vi "ColorSmartCheck.vi"() -> ()   [LabVIEW 2018]
uses:
  <vilib>/myRIO/Instrument Drivers/Onboard IO/AI/typedefs/AI Reference.ctl
  <vilib>/myRIO/Common/Instrument Driver Framework/Utilities/typedefs/myRIO Generic Hardware Reference.ctl
  <vilib>/myRIO/Common/Instrument Driver Framework/Utilities/typedefs/Hardware Version Enum.ctl
  <vilib>/myRIO/Common/Instrument Driver Framework/Utilities/typedefs/myRIO v1.0 Reference.ctl
  <vilib>/myRIO/Common/Instrument Driver Framework/Utilities/typedefs/Generic FPGA Reference.ctl
  <vilib>/myRIO/Common/Instrument Driver Framework/myRIO v1.0/AI/typedefs/AI Channels List.ctl
  <vilib>/myRIO/Common/Instrument Driver Framework/myRIO v1.0/AI/typedefs/AI Channels Enum.ctl
  <vilib>/myRIO/Common/Instrument Driver Framework/Utilities/typedefs/Analog Scaling Constants List.ctl
  <vilib>/myRIO/Common/Instrument Driver Framework/Utilities/typedefs/Analog Scaling Constants.ctl
  <vilib>/userdefined/High Color/nirio_resource_hc.ctl
  <vilib>/Analysis/coordinate.llb/2D Cartesian Coordinate Rotation (Scalar).vi
  <vilib>/Analysis/coordinate.llb/2D Cartesian Coordinate Shift (Scalar).vi
  <vilib>/myRIO/Common/Instrument Driver Framework/Utilities/vis/Is FPGA Ref Available.vi
  <vilib>/myRIO/Common/Instrument Driver Framework/myRIO v1.0/AI/vis/myRIO v1.1 Open AI.vi
  <vilib>/myRIO/Instrument Drivers/Onboard IO/AI/vis/Read.vi
  <vilib>/myRIO/Common/Instrument Driver Framework/Utilities/vis/Validate Channels.vi
  <vilib>/myRIO/Common/Instrument Driver Framework/myRIO v1.0/AI/vis/myRIO v1.0 Reserve AI.vi
  <vilib>/myRIO/Common/Instrument Driver Framework/myRIO v1.0/AI/vis/myRIO v1.0 Build MUX Configuration AI.vi
  <vilib>/myRIO/Common/Instrument Driver Framework/myRIO v1.0/Resource Manager/vis/myRIO v1.0 Reserve Channel List.vi
  <vilib>/myRIO/Common/Instrument Driver Framework/myRIO v1.0/Resource Manager/vis/myRIO v1.0 Reserve Channel.vi
  <vilib>/myRIO/Common/Instrument Driver Framework/myRIO v1.0/Resource Manager/vis/myRIO v1.0 Unreserve Channel.vi
  <vilib>/myRIO/Common/Instrument Driver Framework/myRIO v1.0/Resource Manager/vis/myRIO v1.0 Build Mutex Name.vi
  <vilib>/Utility/VariantDataType/GetNumericInfo.vi
  <vilib>/Utility/error.llb/Error Cluster From Error Code.vi
  <vilib>/myRIO/Common/Instrument Driver Framework/myRIO v1.0/myRIO v1.1 Open.vi
  <vilib>/myRIO/Common/Instrument Driver Framework/myRIO v1.0/AI/vis/myRIO v1.0 Get Scaling Constants AI.vi
  <vilib>/myRIO/Common/Instrument Driver Framework/Utilities/vis/IO Manager.vi
  <vilib>/myRIO/Common/Instrument Driver Framework/Utilities/vis/Configuration Manager.vi
  <vilib>/myRIO/Common/Instrument Driver Framework/myRIO v1.0/myRIO v1.0 Close.vi
  <vilib>/myRIO/Common/Instrument Driver Framework/myRIO v1.0/AI/vis/myRIO v1.0 Read AI.vi
  <vilib>/myRIO/Express VI/Onboard IO/AI/AI Express VI.xnode
  <vilib>/myRIO/Instrument Drivers/Onboard IO/AI/vis/myRIO AI Open.xnode
  <vilib>/myRIO/Instrument Drivers/Onboard IO/AI/AI.lvlib
  <vilib>/Analysis/NI_AALPro.lvlib
panel:
  out "element":string
  out "Found":bool
  out "B/AI0 (Pin 3) 2":dbl
  in  "Theta":dbl
  in  "Right Arm":bool
  in  "Position 2":cluster{"X":dbl, "Y":dbl, "Theta":dbl}
  out "B/AI0 (Pin 3)":dbl
  out "Position":cluster{"X":dbl, "Y":dbl, "Theta":dbl}
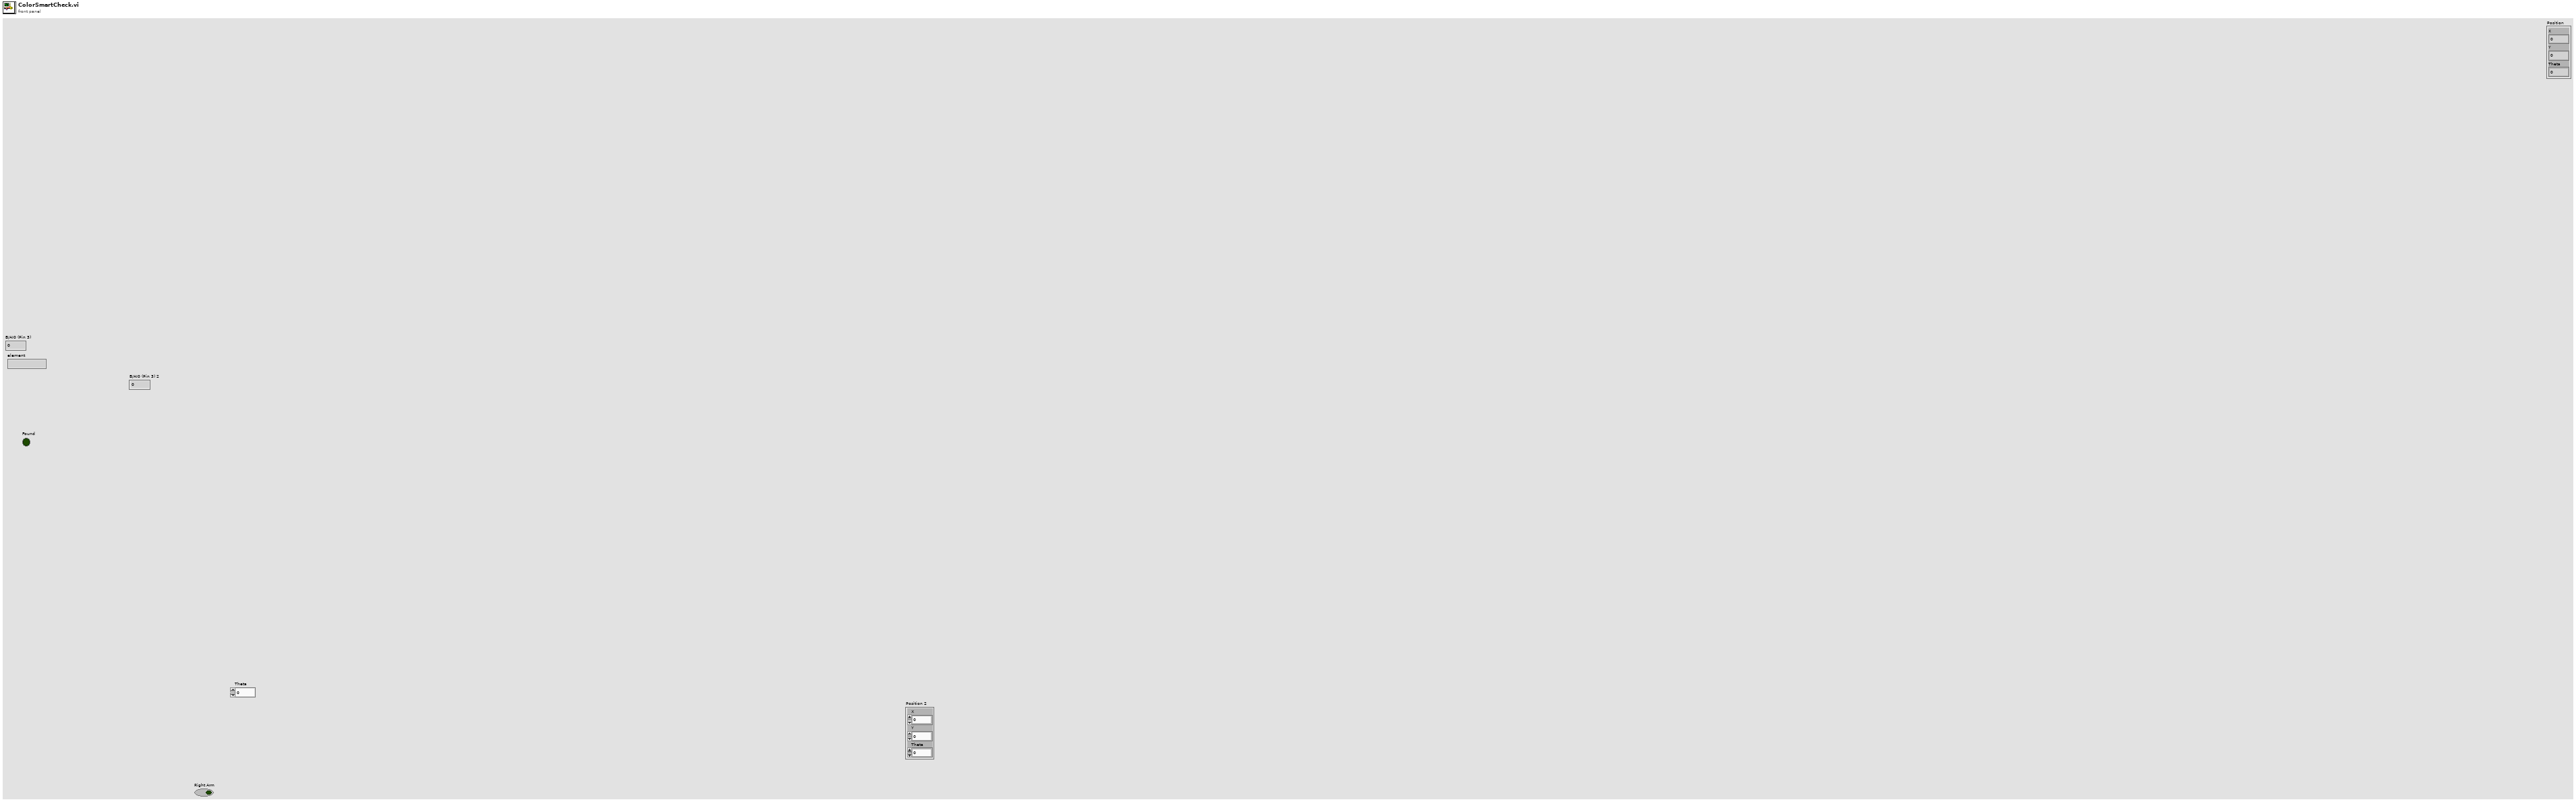
[diagram p1: front panel]
types:
  T1 = typedef "AI.lvlib/AI Reference.ctl" = cluster{"myRIO Reference":T2, "AI Channels List":T6, "AI Scaling Constants List":T8}
  T2 = typedef "myRIO Generic Hardware Reference.ctl" = cluster{"myRIO Model":T3, "myRIO Hardware Reference":T4}
  T3 = typedef "Hardware Version Enum.ctl" = enum16{"Unknown", "myRIO-1900", "myRIO-1950", "roboRIO", "NI ELVIS RIO CM", "ELVIS III"}
  T4 = typedef "myRIO v1.0 Reference.ctl" = cluster{"Generic FPGA Reference":T5, "Allow multiple opens":bool}
  T5 = typedef "Generic FPGA Reference.ctl" = refnum<k20>
  T6 = typedef "AI Channels List.ctl" = T7[]
  T7 = typedef "AI Channels Enum.ctl" = enum16{"Not Connected", "AudioIn/Left", "AudioIn/Right", "C/AI0", "C/AI1", "A/AI0", "A/AI1", "A/AI2", "A/AI3", "A/AI4", "A/AI5", "A/AI6", "A/AI7", "B/AI0", "B/AI1", "B/AI2", "B/AI3", "B/AI4", "B/AI5", "B/AI6", "B/AI7", "AI/AI0", "AI/AI1", "AI/AI2", "AI/AI3", "A/AI0 (DIFF)", "A/AI1 (DIFF)", "A/AI2 (DIFF)", "A/AI3 (DIFF)", "B/AI0 (DIFF)", "B/AI1 (DIFF)", "B/AI2 (DIFF)", "B/AI3 (DIFF)"}
  T8 = typedef "Analog Scaling Constants List.ctl" = T9[]
  T9 = typedef "Analog Scaling Constants.ctl" = cluster{"LSB Weight (Volts)":dbl, "Offset (Volts)":dbl, "Signed?":bool}
  T10 = typedef "nirio_resource_hc.ctl" = tag
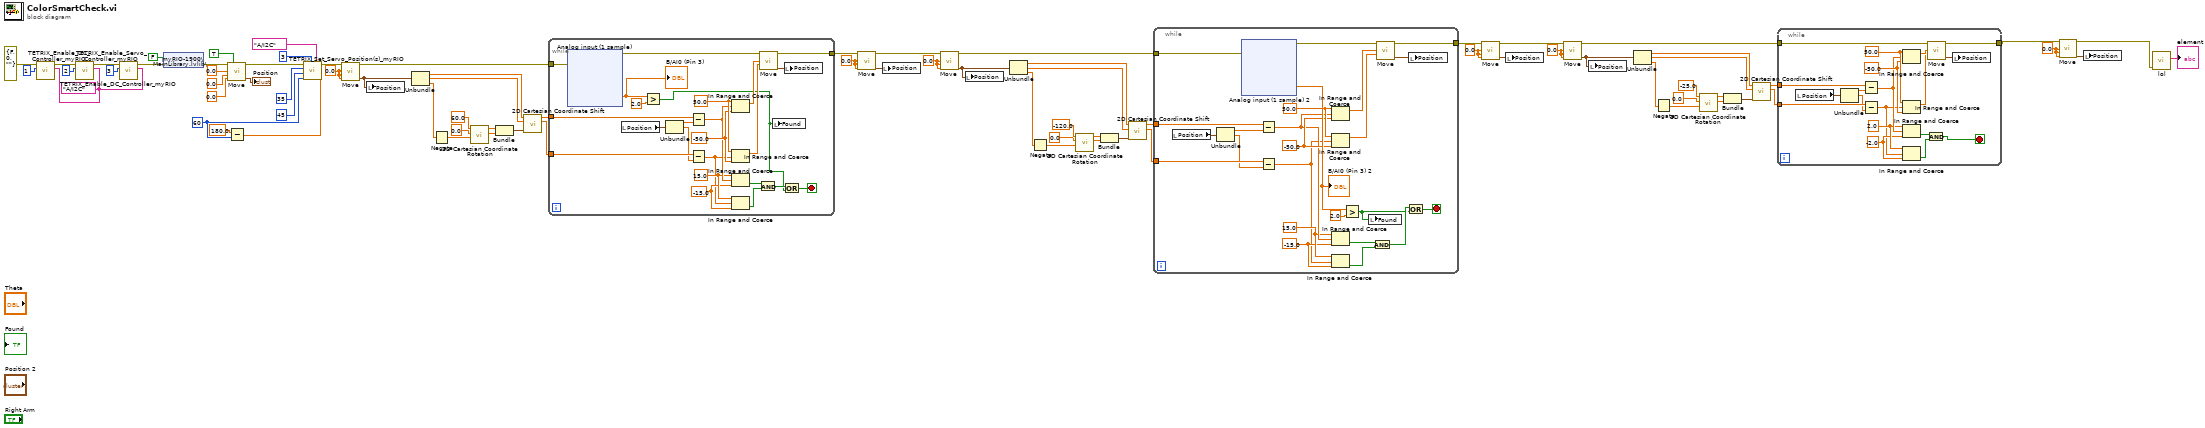
[diagram p0: block diagram]
diagram:
  w5 = 0.0 ("x (mm/s)")
  w12 = 0.0 ("x (mm/s)")
  w23 = 0.0 ("x (mm/s)")
  w31 = 0.0 ("x (mm/s)")
  w54 = 0.0 ("x (mm/s)")
  w46 = 0.0 ("x (mm/s)")
  w57 = tag "A/I2C" ("myRIO MXP Port A/B")
  w73 = u8 60 ("Servo 4 Position (0 - 180 degrees)")
  n1 = call <vilib>:"TETRIX_Enable_DC_Controller_myRIO.vi"("myRIO MXP Port A/B"=w57, "Controller ID#  (I2C Address)"=u8 1, "Error/Flow In"=errorcluster {"status"=FALSE, "code"=0, "source"=""}) -> ("Error/Flow Out"=w61:errorcluster)  [unwired: 4 in]
  n2 = call <vilib>:"TETRIX_Enable_DC_Controller_myRIO.vi"("myRIO MXP Port A/B"=w57, "Controller ID#  (I2C Address)"=u8 2, "Error/Flow In"=w61) -> ("Error/Flow Out"=w63:errorcluster)  [unwired: 4 in]
  n3 = call <vilib>:"TETRIX_Enable_Servo_Controller_myRIO.vi"("myRIO MXP Port A/B"=w57, "Controller ID#  (I2C Address)"=u8 3, "Error/Flow In"=w63) -> ("Error/Flow Out"=w64:errorcluster)  [unwired: 4 in]
  n4 = shared-variable "myRIO-1900\\MainLibrary.lvlib\\stop"(FALSE ("Stop"), error in=w64) -> (error out=w66:errorcluster)
  n5 = call "Move.vi"("Error/Flow In"=w66, "Reset"=TRUE, "x (mm/s)"=0.0, "y (mm/s)"=0.0, "theta (rad/s)"=0.0) -> ("Error/Flow Out"=w78:errorcluster, "Position"=→"Position":cluster{"X":dbl, "Y":dbl, "Theta":dbl})  [unwired: 9 in]
  n6 = Subtract(x=180.0, y=w73) -> (x-y=w74:dbl)
  n7 = call <vilib>:"TETRIX_Set_Servo_Position(s)_myRIO.vi"("Servo 4 Position (0 - 180 degrees)"=w74, "myRIO MXP Port A/B"=tag "A/I2C", "Controller ID#  (I2C Address)"=u8 3, "Servo 3 Position (0 - 180 degrees)"=w73, "Servo 2 Position (0 - 180 degrees)"=u8 45, "Servo 1 Position (0 - 180 degrees)"=u8 35 ("Controller ID#  (I2C Address)"), "Error/Flow In"=w78) -> ("Error/Flow Out"=w45:errorcluster)  [unwired: 2 in]
  n8 = call "Move.vi"("Error/Flow In"=w45, "x (mm/s)"=w46, "y (mm/s)"=w46, "theta (rad/s)"=w46) -> ("Error/Flow Out"=w43:errorcluster, "Position"=w41:cluster{"X":dbl, "Y":dbl, "Theta":dbl})  [unwired: 10 in]
  n9 = local write "Position"(w41) -> ()
  n10 = Unbundle(w41) -> ("X"=w51:dbl, "Y"=w52:dbl, "Theta"=w56:dbl)
  n11 = Negate(x=w56) -> (-x=w55:dbl)
  n12 = call-poly <vilib>:"2D Cartesian Coordinate Rotation.vi"("theta"=w55, "y"=0.0, "x"=60.0) -> ("y out"=w49:dbl, "x out"=w48:dbl)  [unwired: 6 in, 1 out]
  n13 = Bundle("x out"=w48, "y out"=w49) -> (w50:cluster{"x out":dbl, "y out":dbl})  [unwired: 1 in]
  n14 = call-poly <vilib>:"2D Cartesian Coordinate Shift.vi"("shift"=w50, "y"=w52, "x"=w51) -> ("y out"=w39:dbl, "x out"=w40:dbl)  [unwired: 6 in, 1 out]
  n15 = while {
    tunnel: w43 -> [w100]
    tunnel: [w99] -> w42
    tunnel: w40 -> [w97]
    tunnel: w39 -> [w95]
    stop <- w81 stop-if-true
    w86 = -15.0 ("lower limit")
    w87 = 15.0 ("upper limit")
    w91 = -50.0 ("upper limit")
    w92 = 50.0 ("upper limit")
    n16 = xnode "Analog input (1 sample)"("error in (no error)"=w100) -> ("B/AI0 (Pin 3)"=w103:dbl, "error out"=w101:errorcluster)
    "B/AI0 (Pin 3)" <- w103
    n17 = local read "Position"() -> (w98:cluster{"X":dbl, "Y":dbl, "Theta":dbl})
    n18 = Greater?(x=w103, y=2.0) -> (0:w80:bool)
    n19 = Unbundle(w98) -> ("X"=w96:dbl, "Y"=w94:dbl)  [unwired: 1 out]
    n20 = Subtract(x=w97, y=w96) -> (x-y=w88:dbl)
    n21 = Subtract(x=w95, y=w94) -> (x-y=w85:dbl)
    n22 = In Range and Coerce(upper limit=w92, x=w88, lower limit=w91) -> (coerced(x)=w90:dbl)  [unwired: 1 out]
    n23 = In Range and Coerce(upper limit=w92, x=w85, lower limit=w91) -> (coerced(x)=w89:dbl)  [unwired: 1 out]
    n24 = In Range and Coerce(upper limit=w87, x=w88, lower limit=w86) -> (In Range?=w84:bool)  [unwired: 1 out]
    n25 = In Range and Coerce(upper limit=w87, x=w85, lower limit=w86) -> (In Range?=w83:bool)  [unwired: 1 out]
    n26 = And(x=w84, y=w83) -> (x .and. y?=w82:bool)
    n27 = call "Move.vi"("Error/Flow In"=w101, "x (mm/s)"=w90, "y (mm/s)"=w89) -> ("Error/Flow Out"=w99:errorcluster, "Position"=w93:cluster{"X":dbl, "Y":dbl, "Theta":dbl})  [unwired: 11 in]
    n28 = local write "Found"(w80) -> ()
    n29 = Or(x=w82, y=w80) -> (x .or. y?=w81:bool)
    n30 = local write "Position"(w93) -> ()
  }
  n31 = call "Move.vi"("Error/Flow In"=w42, "x (mm/s)"=w54, "y (mm/s)"=w54, "theta (rad/s)"=w54) -> ("Error/Flow Out"=w38:errorcluster, "Position"=w53:cluster{"X":dbl, "Y":dbl, "Theta":dbl})  [unwired: 10 in]
  n32 = local write "Position"(w53) -> ()
  n33 = call "Move.vi"("Error/Flow In"=w38, "x (mm/s)"=w31, "y (mm/s)"=w31, "theta (rad/s)"=w31) -> ("Error/Flow Out"=w33:errorcluster, "Position"=w35:cluster{"X":dbl, "Y":dbl, "Theta":dbl})  [unwired: 10 in]
  n34 = local write "Position"(w35) -> ()
  n35 = Unbundle(w35) -> ("X"=w26:dbl, "Y"=w25:dbl, "Theta"=w21:dbl)
  n36 = Negate(x=w21) -> (-x=w22:dbl)
  n37 = call-poly <vilib>:"2D Cartesian Coordinate Rotation.vi"("theta"=w22, "y"=0.0, "x"=-120.0) -> ("y out"=w28:dbl, "x out"=w29:dbl)  [unwired: 6 in, 1 out]
  n38 = Bundle("x out"=w29, "y out"=w28) -> (w27:cluster{"x out":dbl, "y out":dbl})  [unwired: 1 in]
  n39 = call-poly <vilib>:"2D Cartesian Coordinate Shift.vi"("shift"=w27, "y"=w25, "x"=w26) -> ("y out"=w37:dbl, "x out"=w36:dbl)  [unwired: 6 in, 1 out]
  n40 = while {
    tunnel: w33 -> [w161]
    tunnel: [w160] -> w34
    tunnel: w36 -> [w158]
    tunnel: w37 -> [w156]
    stop <- w142 stop-if-true
    w147 = -15.0 ("lower limit")
    w148 = 15.0 ("upper limit")
    w152 = -50.0 ("upper limit")
    w153 = 50.0 ("upper limit")
    n41 = local read "Position"() -> (w159:cluster{"X":dbl, "Y":dbl, "Theta":dbl})
    n42 = Unbundle(w159) -> ("X"=w157:dbl, "Y"=w155:dbl)  [unwired: 1 out]
    n43 = xnode "Analog input (1 sample) 2"("error in (no error)"=w161) -> ("B/AI0 (Pin 3)"=w164:dbl, "error out"=w162:errorcluster)
    "B/AI0 (Pin 3) 2" <- w164
    n44 = Subtract(x=w158, y=w157) -> (x-y=w149:dbl)
    n45 = Subtract(x=w156, y=w155) -> (x-y=w146:dbl)
    n46 = In Range and Coerce(upper limit=w153, x=w149, lower limit=w152) -> (coerced(x)=w151:dbl)  [unwired: 1 out]
    n47 = In Range and Coerce(upper limit=w153, x=w146, lower limit=w152) -> (coerced(x)=w150:dbl)  [unwired: 1 out]
    n48 = In Range and Coerce(upper limit=w148, x=w149, lower limit=w147) -> (In Range?=w145:bool)  [unwired: 1 out]
    n49 = In Range and Coerce(upper limit=w148, x=w146, lower limit=w147) -> (In Range?=w144:bool)  [unwired: 1 out]
    n50 = Greater?(x=w164, y=2.0) -> (0:w141:bool)
    n51 = local write "Found"(w141) -> ()
    n52 = And(x=w145, y=w144) -> (x .and. y?=w143:bool)
    n53 = call "Move.vi"("Error/Flow In"=w162, "x (mm/s)"=w151, "y (mm/s)"=w150) -> ("Error/Flow Out"=w160:errorcluster, "Position"=w154:cluster{"X":dbl, "Y":dbl, "Theta":dbl})  [unwired: 11 in]
    n54 = Or(x=w143, y=w141) -> (x .or. y?=w142:bool)
    n55 = local write "Position"(w154) -> ()
  }
  n56 = call "Move.vi"("Error/Flow In"=w34, "x (mm/s)"=w23, "y (mm/s)"=w23, "theta (rad/s)"=w23) -> ("Error/Flow Out"=w9:errorcluster, "Position"=w24:cluster{"X":dbl, "Y":dbl, "Theta":dbl})  [unwired: 10 in]
  n57 = local write "Position"(w24) -> ()
  n58 = call "Move.vi"("Error/Flow In"=w9, "x (mm/s)"=w12, "y (mm/s)"=w12, "theta (rad/s)"=w12) -> ("Error/Flow Out"=w6:errorcluster, "Position"=w10:cluster{"X":dbl, "Y":dbl, "Theta":dbl})  [unwired: 10 in]
  n59 = local write "Position"(w10) -> ()
  n60 = Unbundle(w10) -> ("X"=w17:dbl, "Y"=w18:dbl, "Theta"=w20:dbl)
  n61 = Negate(x=w20) -> (-x=w19:dbl)
  n62 = call-poly <vilib>:"2D Cartesian Coordinate Rotation.vi"("theta"=w19, "y"=0.0, "x"=-25.0) -> ("y out"=w15:dbl, "x out"=w14:dbl)  [unwired: 6 in, 1 out]
  n63 = Bundle("x out"=w14, "y out"=w15) -> (w16:cluster{"x out":dbl, "y out":dbl})  [unwired: 1 in]
  n64 = call-poly <vilib>:"2D Cartesian Coordinate Shift.vi"("shift"=w16, "y"=w18, "x"=w17) -> ("y out"=w7:dbl, "x out"=w8:dbl)  [unwired: 6 in, 1 out]
  n65 = while {
    tunnel: [w220] -> w3
    tunnel: w8 -> [w218]
    tunnel: w7 -> [w216]
    tunnel: w6 -> [w203]
    stop <- w202 stop-if-true
    w207 = -2.0 ("lower limit")
    w208 = 2.0 ("upper limit")
    w212 = -50.0 ("upper limit")
    w213 = 50.0 ("upper limit")
    n66 = local read "Position"() -> (w219:cluster{"X":dbl, "Y":dbl, "Theta":dbl})
    n67 = Unbundle(w219) -> ("X"=w217:dbl, "Y"=w215:dbl)  [unwired: 1 out]
    n68 = Subtract(x=w218, y=w217) -> (x-y=w209:dbl)
    n69 = Subtract(x=w216, y=w215) -> (x-y=w206:dbl)
    n70 = In Range and Coerce(upper limit=w213, x=w209, lower limit=w212) -> (coerced(x)=w211:dbl)  [unwired: 1 out]
    n71 = In Range and Coerce(upper limit=w213, x=w206, lower limit=w212) -> (coerced(x)=w210:dbl)  [unwired: 1 out]
    n72 = In Range and Coerce(upper limit=w208, x=w209, lower limit=w207) -> (In Range?=w205:bool)  [unwired: 1 out]
    n73 = In Range and Coerce(upper limit=w208, x=w206, lower limit=w207) -> (In Range?=w204:bool)  [unwired: 1 out]
    n74 = And(x=w205, y=w204) -> (x .and. y?=w202:bool)
    n75 = call "Move.vi"("Error/Flow In"=w203, "x (mm/s)"=w211, "y (mm/s)"=w210) -> ("Error/Flow Out"=w220:errorcluster, "Position"=w214:cluster{"X":dbl, "Y":dbl, "Theta":dbl})  [unwired: 11 in]
    n76 = local write "Position"(w214) -> ()
  }
  n77 = call "Move.vi"("Error/Flow In"=w3, "x (mm/s)"=w5, "y (mm/s)"=w5, "theta (rad/s)"=w5) -> ("Error/Flow Out"=w1:errorcluster, "Position"=w4:cluster{"X":dbl, "Y":dbl, "Theta":dbl})  [unwired: 10 in]
  n78 = local write "Position"(w4) -> ()
  n79 = call "lol.vi"("error in"=w1) -> ("element"=→"element":string)  [unwired: 9 in, 1 out]
